vi "Remove Topic.vi"(8 "error in (no error)":errorcluster, 10 "Topic Name":string, 11 "TopicLookupTable in":refnum<class "TopicLookupTable.lvclass">) -> (0 "error out":errorcluster, 3 "TopicLookupTable out":refnum<class "TopicLookupTable.lvclass">)   [LabVIEW 2015, in "Mediator.lvlib" / "TopicLookupTable.lvclass"]
uses:
  TopicLookupTable.lvclass
  TopicLookupTable.lvclass/TopicLookupTable.ctl
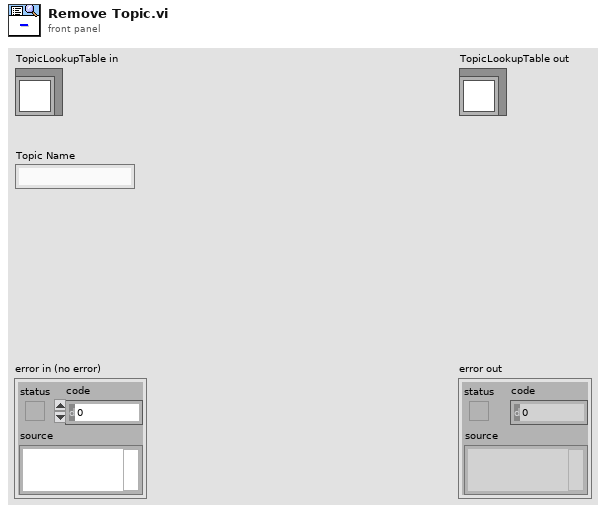
[diagram p1: front panel]
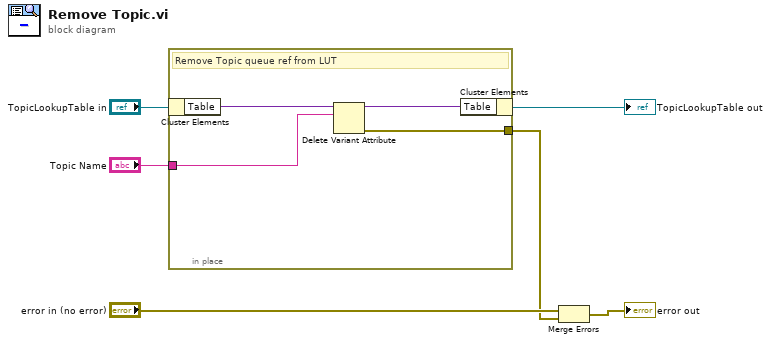
[diagram p0: block diagram]
diagram:
  n1 = in-place {
    in-place-border: [w8] -> w2
    in-place-border: "Topic Name" -> [w7]
    # "Remove Topic queue ref from LUT"
    n2 = in-place-cluster #1("TopicLookupTable in") -> ("Table"=w10:variant)
    n3 = Delete Variant Attribute(6:w7, 7:w10) -> (0:w8:errorcluster, 3:w9:variant)  [unwired: 1 in, 1 out]
    n4 = in-place-cluster #1("Table"=w9) -> (→"TopicLookupTable out":refnum<class "TopicLookupTable.lvclass">)
  }
  n5 = Merge Errors("error in (no error)", w2) -> (→"error out":errorcluster)
